vi "Get Perspective Transform.vi"(8 "error in (no error)":errorcluster, 10 "To":T1, 11 "From":T1) -> (0 "error out":errorcluster, 3 "3x3 Warp Matrix":T3)   [LabVIEW 2020, in "image.lvlib"]
doc: "Compute the perspective transform which maps the From-Points to the To-Points."
uses:
  image.lvlib
  <vilib>/Analysis/Matrix/Datatypes/RealMatrix.ctl
  common/Image Points Quad (Float).ctl
  common/Image Point (Float).ctl
  Matrix(3x3).ctl
  Vector(3 Element).ctl
  <vilib>/Analysis/Matrix/Numeric/Conversions/Array To Matrix - RA2.vi
  common/common.lvlib
  <vilib>/Analysis/Matrix/NI_Matrix.lvlib
  common/bin/gartoolkit_32-1.dll
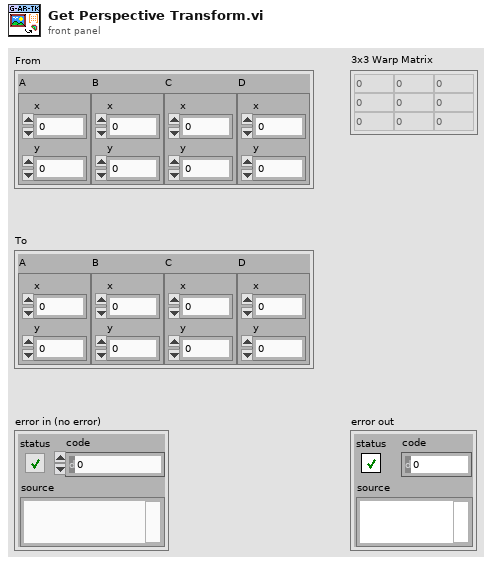
[diagram p1: front panel]
types:
  T1 = typedef "common.lvlib/Image Points Quad (Float).ctl" = cluster{"A":T2, "B":T2, "C":T2, "D":T2}
  T2 = typedef "common.lvlib/Image Point (Float).ctl" = cluster{"x":dbl, "y":dbl}
  T3 = typedef "NI_Matrix.lvlib/RealMatrix.ctl" = dbl[][]
  T4 = typedef "image.lvlib/Matrix(3x3).ctl" = cluster{"0":T5, "1":T5, "2":T5}
  T5 = typedef "image.lvlib/Vector(3 Element).ctl" = cluster{"0":dbl, "1":dbl, "2":dbl}
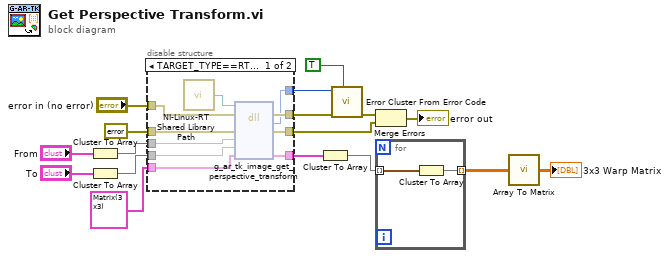
[diagram p0: block diagram]
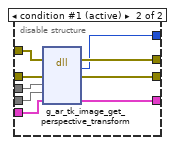
[diagram p2: hidden frame]
diagram:
  n1 = Cluster To Array(cluster="From") -> (array=w8:T2[])
  n2 = Cluster To Array(cluster="To") -> (array=w6:T2[])
  n3 = disable-structure shown="TARGET_TYPE==RT&&OS==Linux" {
    disable-tunnel: "error in (no error)" -> [w27 w36]
    disable-tunnel: errorcluster {"status"=FALSE, "code"=0, "source"=""} ("error constant") -> [w26 w35]
    disable-tunnel: [w22 w34] -> w13
    disable-tunnel: [w21 w33] -> w14
    disable-tunnel: [w20 w32] -> w15
    disable-tunnel: T4 {"0"={"0"=0.0, "1"=0.0, "2"=0.0}, "1"={"0"=0.0, "1"=0.0, "2"=0.0}, "2"={"0"=0.0, "1"=0.0, "2"=0.0}} ("Matrix out") -> [w23 w29]
    disable-tunnel: w8 -> [w25 w31]
    disable-tunnel: w6 -> [w24 w30]
    disable-tunnel: [w18 w28] -> w5
    frame condition #0 {
      n4 = call "NI-Linux-RT Shared Library Path.vi"() -> ("Path"=w19:path)
      n5 = dll-call lib="?" fn="g_ar_tk_image_get_perspective_transform" ("g_ar_toolkit.*.*:g_ar_tk_image_warp_perspective")(path in=w19, error in=w27, "error_cluster"=w26, "Points A"=w25, "Points B"=w24, "matrix"=w23) -> (error out=w22:errorcluster, w21:i32, "error_cluster"=w20:errorcluster, "matrix"=w18:T4)  [unwired: 3 in, 1 out]
    }
    frame condition #1 (active) {
      n6 = dll-call lib="C:/serenial/lib/g-augmented-reality-toolkit/LabVIEW/common/bin/gartoolkit_*-1.*" fn="g_ar_tk_image_get_perspective_transform" ("g_ar_toolkit.*.*:g_ar_tk_image_warp_perspective")(error in=w36, "error_cluster"=w35, "Points A"=w31, "Points B"=w30, "matrix"=w29) -> (error out=w34:errorcluster, w33:i32, "error_cluster"=w32:errorcluster, "matrix"=w28:T4)  [unwired: 4 in, 1 out]
    }
  }
  n7 = Cluster To Array(cluster=w5) -> (array=w4:T5[])
  n8 = call <vilib>:"Error Cluster From Error Code.vi"("show call chain? (False)"=TRUE, "error in (no error)"=w13, "error code (0)"=w14) -> ("error out"=w11:errorcluster)  [unwired: 6 in]
  n9 = Merge Errors(w11, w15) -> (→"error out":errorcluster)
  n10 = for {
    tunnel: w4 -> [w38] mode=indexing
    tunnel: [w37] -> w3 mode=indexing
    n11 = Cluster To Array(cluster=w38) -> (array=w37:dbl[])
  }
  n12 = call-poly <vilib>:"Array To Matrix.vi"("Real 2D Array"=w3) -> ("Real Matrix"=→"3x3 Warp Matrix":T3)
